vi "ble_cmd_sm_delete_bonding.vi"(8 "error in (no error)":errorcluster, 10 "Bonding Handle (0xFF = all)":u8=255 format="%02x", 11 "COM Bluegiga in":refnum<visa-resource-name>) -> (0 "error out":errorcluster, 3 "COM Bluegiga out":refnum<visa-resource-name>)   [LabVIEW 2015]
uses:
  <vilib>/BLE/type_def/message_class.ctl
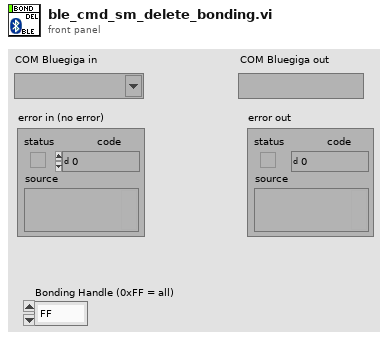
[diagram p1: front panel]
types:
  T1 = typedef "message_class.ctl" = u8
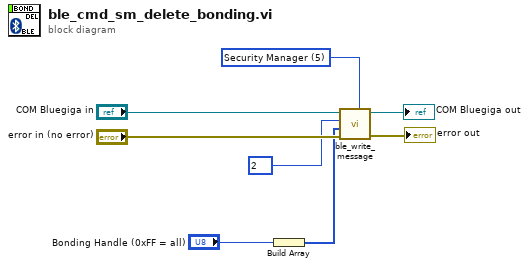
[diagram p0: block diagram]
diagram:
  w4 = T1 5 items=["System", "Persistent Store", "Attribute database", "Connection", "Attribute client", "Security Manager", "Generic Access Profile", "Hardware"] ("Command Class (System)")
  n1 = Build Array("Bonding Handle (0xFF = all)") -> (w5:u8[])
  n2 = call <vilib>:"ble_write_message.vi"("Command Class (System)"=w4, "error in (no error)"="error in (no error)", "Payload(Empty)"=w5, "Message ID (0x00)"=u8 2, "COM Bluegiga in"="COM Bluegiga in") -> ("error out"=→"error out":errorcluster, "COM Bluegiga out"=→"COM Bluegiga out":refnum<visa-resource-name>)  [unwired: 4 in, 1 out]
